vi "Draw Text to Image.vi"(9 "BG Color":u32(colorbox)=5789784, 10 "Text":string, 11 "Refnum in":T1) -> (3 "Refnum out":T1)   [LabVIEW 2016]
uses:
  <vilib>/vision/Image Controls.llb/IMAQ Image.ctl
  <vilib>/vision/NI_Vision_Development_Module.lvlib
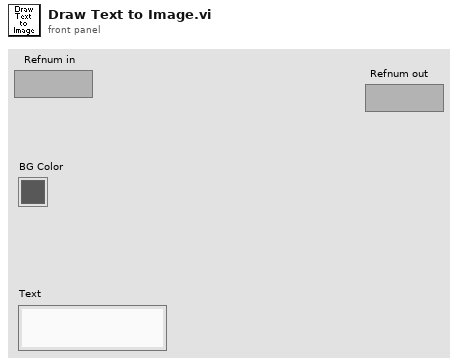
[diagram p1: front panel]
types:
  T1 = typedef "IMAQ Image.ctl" = refnum<image>
  T2 = cluster{"Desired Font (Application)":enum16{"User-specified Font", "Application Font", "System Font", "Dialog Font"}, "[User-specified Font]":cluster{"Font Name":string, "Size":i16, "Strikeout?":bool, "Italic?":bool, "Underline?":bool, "Outline?":bool, "Shadow?":bool, "Bold?":bool, "Rotation Angle":dbl}, "Horizontal Alignment":i16, "Vertical Alignment":i16}
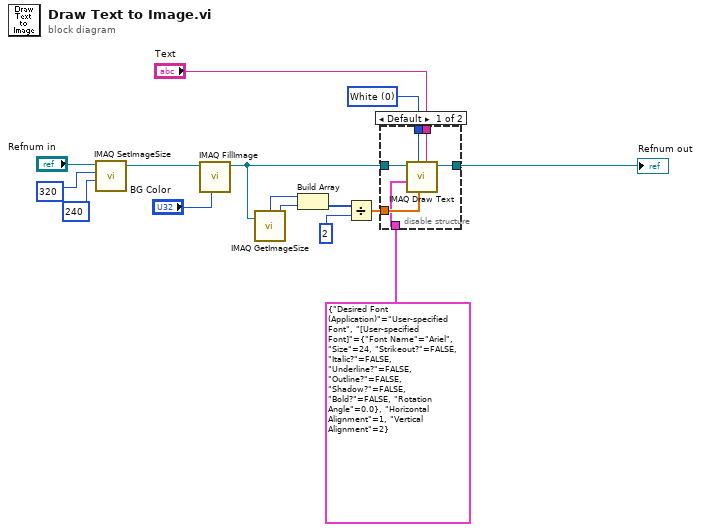
[diagram p0: block diagram]
diagram:
  w12 = 0 items=["White", "Black", "Inverted", "Black on White", "White on Black"] ("Color")
  n1 = call "IMAQ SetImageSize"("Y Resolution"=240, "X Resolution"=320, "Image"="Refnum in") -> ("Image Out"=w3:T1)  [unwired: 2 in, 1 out]
  n2 = call "IMAQ FillImage"("Color Pixel Value"="BG Color", "Image"=w3) -> ("Image Out"=w10:T1)  [unwired: 8 in, 1 out]
  n3 = call "IMAQ GetImageSize"("Image"=w10) -> ("Y Resolution"=w7:i32, "X Resolution"=w8:i32)  [unwired: 3 in, 1 out]
  n4 = Build Array(w8, w7) -> (w6:i32[])
  n5 = Divide(x=w6, y=2) -> (x/y=w5:dbl[])
  n6 = disable-structure shown="Default" {
    disable-tunnel: [w20 _] -> w14
    disable-tunnel: "Text" -> [w19 _]
    disable-tunnel: w12 -> [w18 _]
    disable-tunnel: T2 {"Desired Font (Application)"=enum."User-specified Font", "[User-specified Font]"={"Font Name"="Ariel", "Size"=24, "Strikeout?"=FALSE, "Italic?"=FALSE, "Underline?"=FALSE, "Outline?"=FALSE, "Shadow?"=FALSE, "Bold?"=FALSE, "Rotation Angle"=0.0}, "Horizontal Alignment"=1, "Vertical Alignment"=2} ("Font, Size & Style") -> [w16 _]
    disable-tunnel: w10 -> [w21 _]
    disable-tunnel: w5 -> [w17 _]
    frame condition #0 (active) {
      n7 = call "IMAQ Draw Text"("String"=w19, "Insertion Point"=w17, "Color"=w18, "Font, Size & Style"=w16, "Image Src"=w21) -> ("Image Dst Out"=w20:T1)  [unwired: 3 in, 3 out]
    }
    frame condition #1 {
    }
  }
  "Refnum out" <- w14
